vi "initialize.vi"(0 "HGF_FGV_SelectionByName":refnum<class "HGF_FGV_SelectByName.lvclass">, 3 "initializationData":variant, 5 "error in (no error)":errorcluster, 7 "binaryString":string, 8 "I8 Array":i8[](array[numeric]), 9 "prependSize? (T)":bool, 11 "byteOrder (0:big-endian, network order)":T1(ring)) -> (14 "dup HGF_FGV_SelectionByName":refnum<class "HGF_FGV_SelectByName.lvclass">, 17 "found?":bool, 19 "error out":errorcluster)   [LabVIEW 2012, in "HGF_FGV.lvlib" / "HGF_FGV_SelectByName.lvclass"]
doc: "This is a dynamic dispatch VI to be implemented by child classes to initialize their attributes.\n\n<B>Attention:</B> Support for Variant for initialization data only."
uses:
  HGF_FGV_SelectByName.lvclass
  HGF_FGV_Action/HGF_FGV_Action.lvclass
  HGF_FGV_SelectByName.lvclass/HGF_FGV_SelectByName.ctl
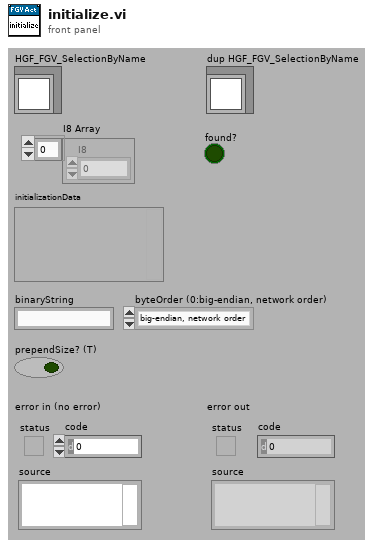
[diagram p1: front panel]
types:
  T1 = enum16{"big-endian, network order", "native, host order", "little-endian"}
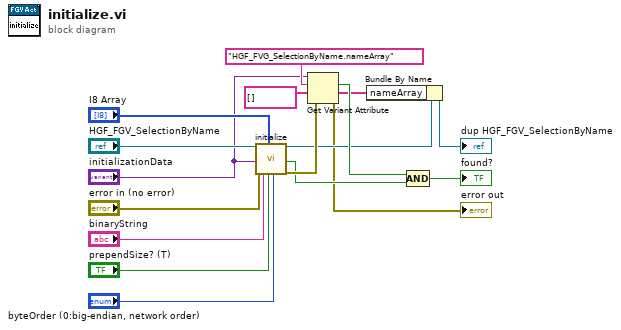
[diagram p0: block diagram]
diagram:
  n1 = call-parent "initialize.vi"("HGF_Factory"="HGF_FGV_SelectionByName", "initializationData"="initializationData", "error in (no error)"="error in (no error)", "binaryString"="binaryString", "I8 Array"="I8 Array", "prependSize? (T)"="prependSize? (T)", "byteOrder (0:big-endian, network order)"="byteOrder (0:big-endian, network order)") -> ("dup HGF_Factory"=w8:refnum<class "HGF_FGV_SelectByName.lvclass">, "found?"=w13:bool, "error out"=w14:errorcluster)  [unwired: 1 in, 9 out]
  n2 = Get Variant Attribute(Variant="initializationData", name="HGF_FVG_SelectionByName.nameArray", default value (empty Variant)=string[] [] ("nameArray"), error in=w14) -> (found=w9:bool, value=w5:string[], error out=→"error out":errorcluster)  [unwired: 1 out]
  n3 = Bundle By Name(cluster=w8, "nameArray"=w5) -> (→"dup HGF_FGV_SelectionByName":refnum<class "HGF_FGV_SelectByName.lvclass">)
  n4 = Compound Arithmetic op=AND(w9, w13) -> (→"found?":bool)
